vi "Read.vi"(8 "error in":errorcluster, 11 "Chiller Cluster.lvclass":refnum<class "Chiller Cluster.lvclass">) -> (0 "error out":errorcluster, 1 "Channels":T1(array[cluster]), 2 "Controls":T2, 3 "output cluster":refnum<class "Chiller Cluster.lvclass">)   [LabVIEW 2023, in "Chiller Cluster.lvclass"]
uses:
  Chiller Cluster.lvclass
  Chiller Cluster.lvclass/Chiller Cluster.ctl
  c513e7c0-ccb2-43ae-9fd9-aade89634a4e.vi
  1a9b8b61-8a11-41d6-bef0-d3d32e632910.vi
  c513e7c0-ccb2-43ae-9fd9-aade89634a4e.vi/c28b0ead-42ad-4072-80a2-aca7f2bd7ce3.vi
  c513e7c0-ccb2-43ae-9fd9-aade89634a4e.vi/219d0231-d98b-4193-b5cc-84f90e3c9091.vi
  1a9b8b61-8a11-41d6-bef0-d3d32e632910.vi/c28b0ead-42ad-4072-80a2-aca7f2bd7ce3.vi
  1a9b8b61-8a11-41d6-bef0-d3d32e632910.vi/219d0231-d98b-4193-b5cc-84f90e3c9091.vi
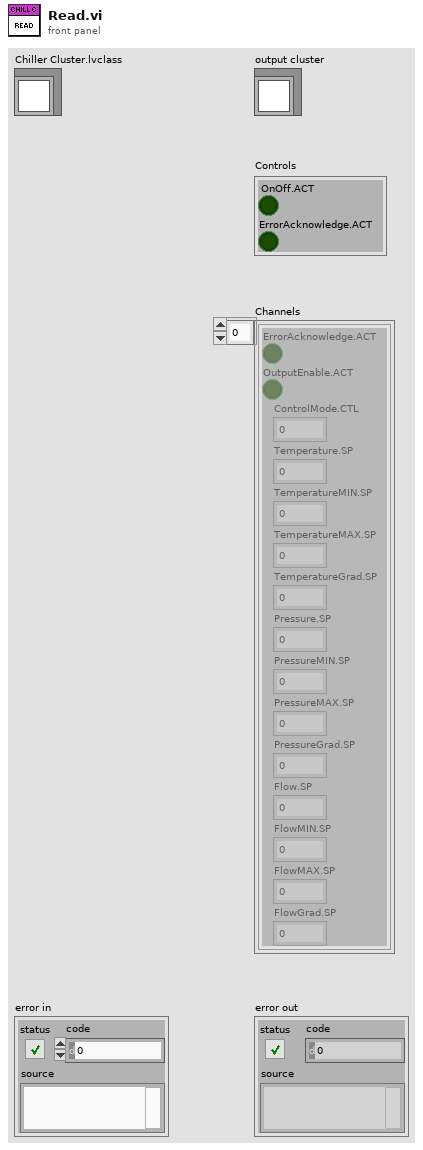
[diagram p1: front panel]
types:
  T1 = cluster{"ErrorAcknowledge.ACT":bool, "OutputEnable.ACT":bool, "ControlMode.CTL":u16, "Temperature.SP":dbl, "TemperatureMIN.SP":dbl, "TemperatureMAX.SP":dbl, "TemperatureGrad.SP":dbl, "Pressure.SP":dbl, "PressureMIN.SP":dbl, "PressureMAX.SP":dbl, "PressureGrad.SP":dbl, "Flow.SP":dbl, "FlowMIN.SP":dbl, "FlowMAX.SP":dbl, "FlowGrad.SP":dbl}[]
  T2 = cluster{"OnOff.ACT":bool, "ErrorAcknowledge.ACT":bool}
  T3 = cluster{"ErrorAcknowledge.ACT":bool, "OutputEnable.ACT":bool, "ControlMode.CTL":u16, "Temperature.SP":dbl, "TemperatureMIN.SP":dbl, "TemperatureMAX.SP":dbl, "TemperatureGrad.SP":dbl, "Pressure.SP":dbl, "PressureMIN.SP":dbl, "PressureMAX.SP":dbl, "PressureGrad.SP":dbl, "Flow.SP":dbl, "FlowMIN.SP":dbl, "FlowMAX.SP":dbl, "FlowGrad.SP":dbl}
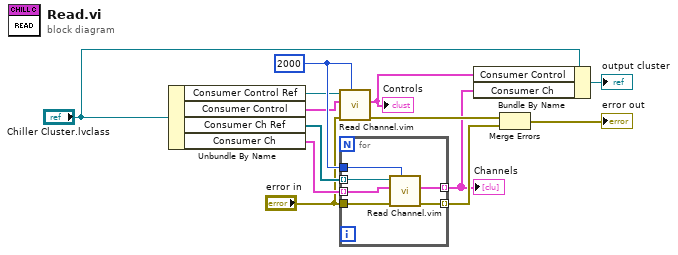
[diagram p0: block diagram]
diagram:
  w13 = 2000 ("Timeout (ms)")
  n1 = Unbundle By Name("Chiller Cluster.lvclass") -> ("Consumer Control Ref"=w12:refnum<k21>, "Consumer Control"=w11:T2, "Consumer Ch Ref"=w10:refnum<k21>[], "Consumer Ch"=w9:T1)
  n2 = call "Read Channel.vim"("Timeout (ms)"=w13, "error in"="error in", "Data in"=w11, "ADAS HIL Channel in"=w12) -> ("error out"=w5:errorcluster, "Data out"=w2:T2)  [unwired: 4 in, 2 out]
  "Controls" <- w2
  n3 = for {
    tunnel: w13 -> [w19]
    tunnel: w10 -> [w18] mode=indexing
    tunnel: w9 -> [w17] mode=indexing
    tunnel: "error in" -> [w16]
    tunnel: [w15] -> w1 mode=indexing
    tunnel: [w14] -> w6 mode=indexing
    n4 = call "Read Channel.vim"("Timeout (ms)"=w19, "error in"=w16, "Data in"=w17, "ADAS HIL Channel in"=w18) -> ("error out"=w14:errorcluster, "Data out"=w15:T3)  [unwired: 4 in, 2 out]
  }
  "Channels" <- w1
  n5 = Bundle By Name(cluster="Chiller Cluster.lvclass", "Consumer Control"=w2, "Consumer Ch"=w1) -> (→"output cluster":refnum<class "Chiller Cluster.lvclass">)
  n6 = Merge Errors(w5, w6) -> (→"error out":errorcluster)
